vi "Angle U to Deg.vi"(10 "Angle U zero":dbl, 11 "Angle U":dbl) -> (2 "Angle U":dbl, 3 "Angle":dbl)   [LabVIEW 2019, in "DAC.lvlib" / "DAC Inclinometer.lvclass"]
uses:
  DAC Inclinometer.lvclass
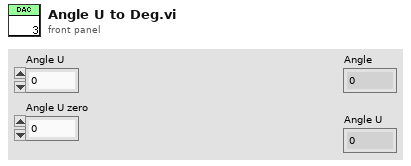
[diagram p1: front panel]
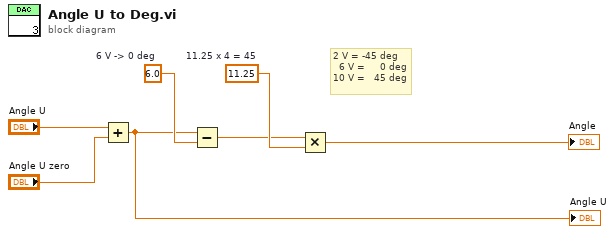
[diagram p0: block diagram]
diagram:
  w4 = 6.0  # 6 V -> 0 deg
  w7 = 11.25  # 11.25 x 4 = 45
  # "2 V = -45 deg\n  6 V =     0 deg\n10 V =   45 deg"
  n1 = Add(x="Angle U", y="Angle U zero") -> (x+y=w3:dbl)
  "Angle U" <- w3
  n2 = Subtract(x=w3, y=w4) -> (x-y=w2:dbl)
  n3 = Multiply(x=w2, y=w7) -> (x*y=→"Angle":dbl)
